vi "configure operation.vi"(7 "Shared Library Module configuration in":refnum<class "Shared Library Module configuration.lvclass">, 8 "error in":errorcluster, 10 "line item in":T1, 11 "engine configuration in":refnum<class "engine configuration.lvclass">) -> (0 "error out":errorcluster, 1 "success":bool, 2 "line item out":T1, 5 "changed":bool)   [LabVIEW 2013, in "Shared Library Module editor node.lvclass"]
doc: "Platypus Framework 1.0.1.60\nNI Systems Engineering - National Instruments"
uses:
  Shared Library Module editor node.lvclass
  permissions.ctl
  table line.ctl
  <vilib>/NI/Tag Bus Module Framework/channel/TBM channel.lvclass
  <vilib>/NI/Module Execution Interface/Engine Configuration/engine configuration.lvclass
  configuration/Shared Library Module configuration.lvclass
  <vilib>/NI/Configuration Framework/serializable configuration/NISE_CEF_serializable configuration.lvclass/NISE_CEF_serializable configuration.ctl
  <vilib>/NI/Tag Bus Module Framework/channel/TBM channel.lvclass/TBM channel.ctl
  <vilib>/NI/Tag Bus/tag/tag descriptor.lvclass/tag descriptor.ctl
  <vilib>/NI/Configuration Framework/serializable configuration/Read UID.vi
  <vilib>/NI/Tag Bus Module Framework/channel/Read channel classification.vi
  <vilib>/NI/Tag Bus/tag/read data type.vi
  <vilib>/NI/Tag Bus/tag/write tag name.vi
  <vilib>/NI/Tag Bus/tag/write data type.vi
  <vilib>/NI/Tag Bus Module Framework/channel/Write channel classification.vi
  <vilib>/Utility/LVClass/Get LV Class Name.vi
  <vilib>/NI/Configuration Framework/error generator/NISE_error generator.vi
  <vilib>/NI/Tag Bus/tag/tag descriptor.lvclass
panel:
  in  "Tag":i32(listbox)
  in  "Type":i32(listbox)
  in  "Channel Name":string
  in  "cancel":bool
  in  "ok":bool
  in  "Access Type":T2
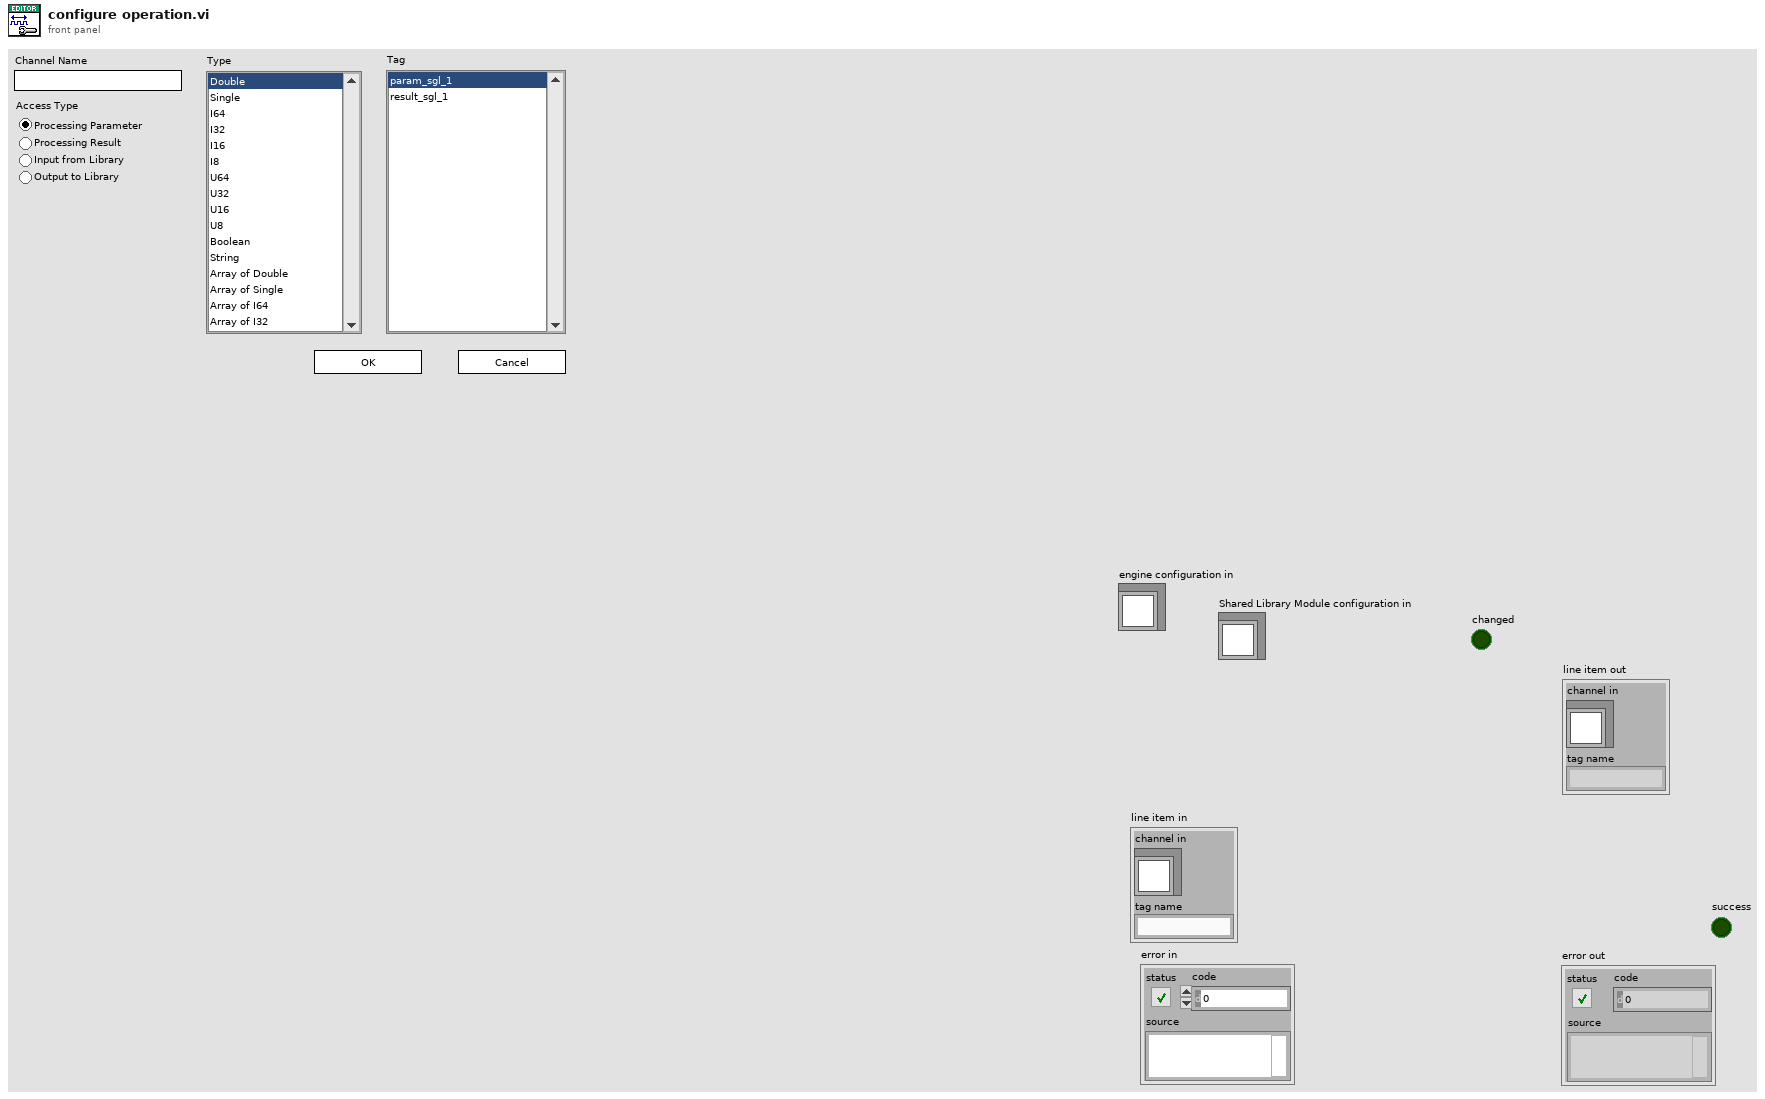
[diagram p1: front panel]
types:
  T1 = typedef "Shared Library Module editor node.lvclass/table line.ctl" = cluster{"channel in":refnum<class "TBM channel.lvclass">, "tag name":string}
  T2 = typedef "Shared Library Module editor node.lvclass/permissions.ctl" = enum32{"Processing Parameter", "Processing Result", "Input from Library", "Output to Library"}
  T3 = enum32{"Invalid", "Standard", "Closed", "Hidden", "Minimized", "Maximized"}
  T4 = enum32{"Invalid", "Default", "Floating", "Floating/Auto-Hide", "Modal"}
  T5 = enum8{"Enabled", "Disabled", "Disabled and Grayed Out"}
  T6 = typedef "tag bus.lvlib/tag descriptor.lvclass/Data Type.ctl" = enum16{"Double", "Single", "I64", "I32", "I16", "I8", "U64", "U32", "U16", "U8", "Boolean", "String", "Array of Double", "Array of Single", "Array of I64", "Array of I32", "Array of I16", "Array of I8", "Array of U64", "Array of U32", "Array of U16", "Array of U8", "Array of Boolean", "Array of String"}
  T7 = enum32{"invalid app kind", "Development System", "Run Time System", "Student Edition", "Embedded LabVIEW", "Evaluation", "Custom"}
  T8 = typedef "TBM channel.lvclass/channel classification.ctl" = enum16{"input data", "output data", "processing parameter", "processing result"}
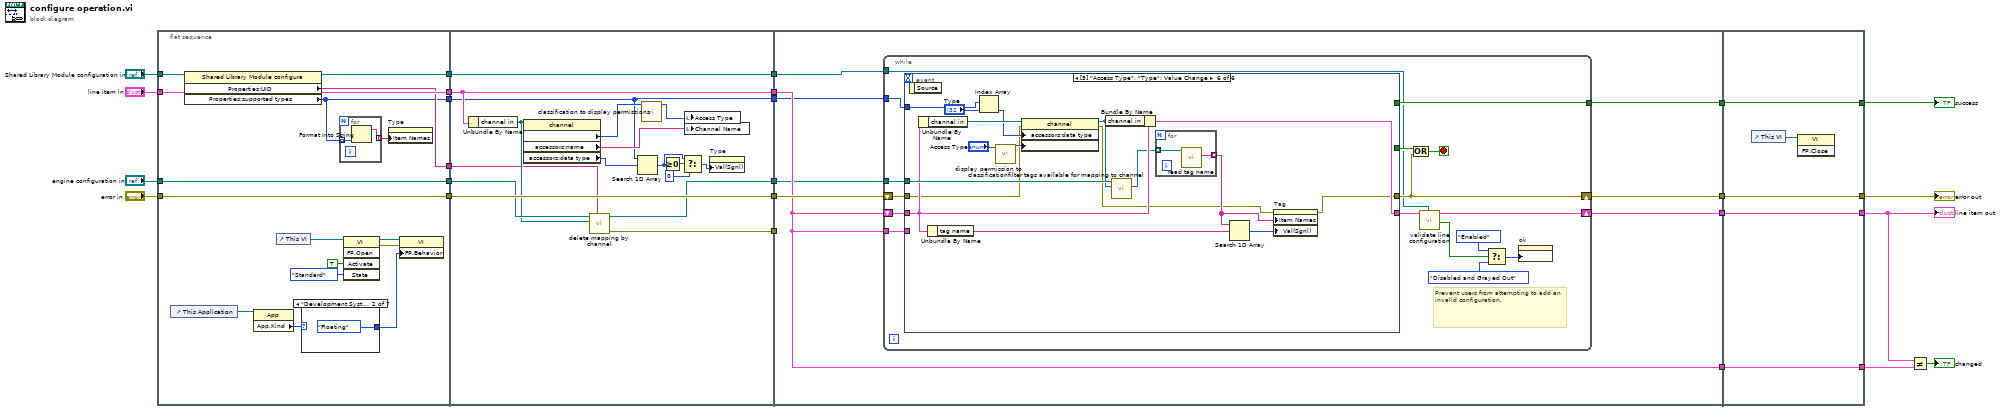
[diagram p0: block diagram]
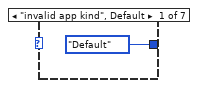
[diagram p2: hidden frame]
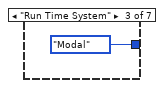
[diagram p3: hidden frame]
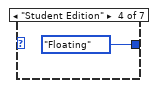
[diagram p4: hidden frame]
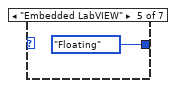
[diagram p5: hidden frame]
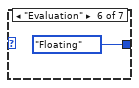
[diagram p6: hidden frame]
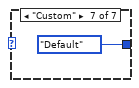
[diagram p7: hidden frame]
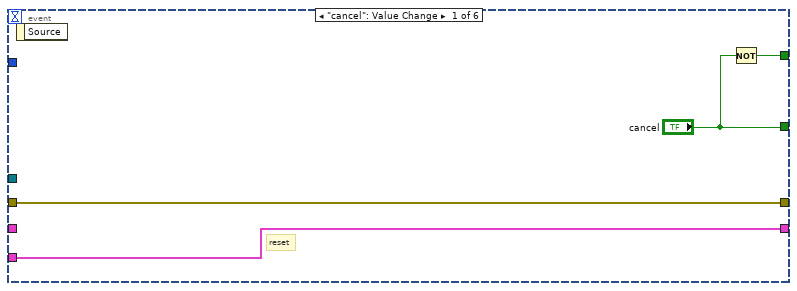
[diagram p8: hidden frame]
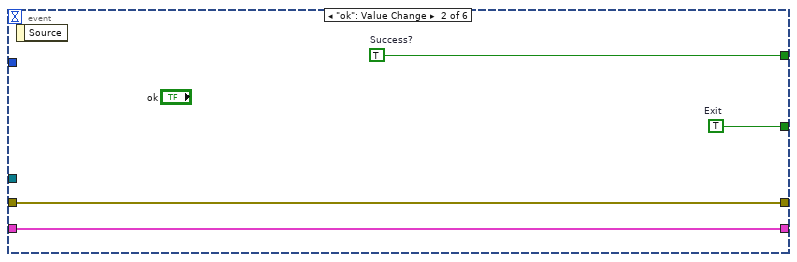
[diagram p9: hidden frame]
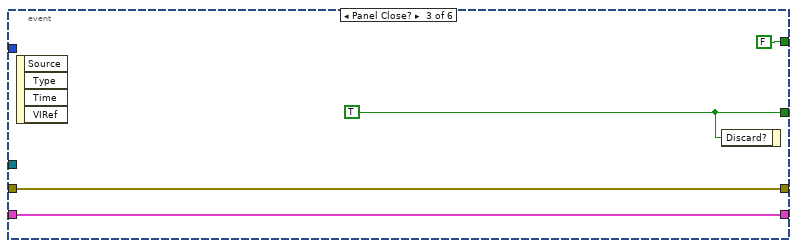
[diagram p10: hidden frame]
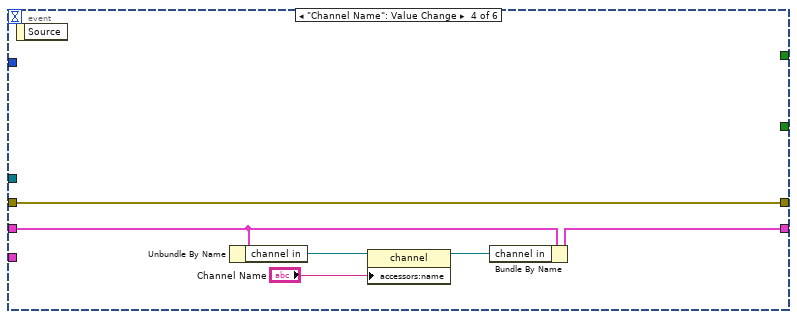
[diagram p11: hidden frame]
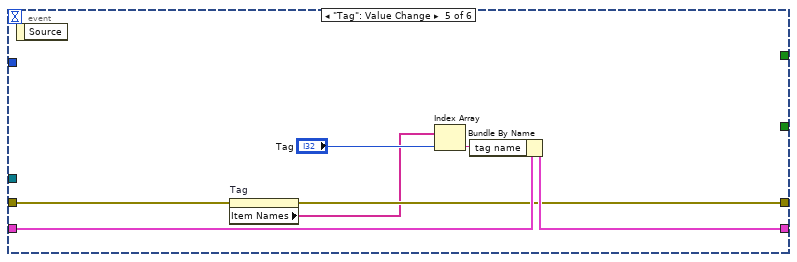
[diagram p12: hidden frame]
diagram:
  n1 = flat-sequence {
    tunnel: "line item in" -> [w40]
    tunnel: "error in" -> [w41]
    tunnel: [w41] -> w14
    tunnel: [w40] -> w12
    tunnel: [w29] -> w10
    tunnel: "Shared Library Module configuration in" -> [w31]
    tunnel: "engine configuration in" -> [w30]
    tunnel: [w30] -> w6
    tunnel: [w28] -> w4
    tunnel: [w27] -> w3
    tunnel: w14 -> [w67]
    tunnel: [w67] -> w13
    tunnel: w12 -> [w63]
    tunnel: [w63] -> w11
    tunnel: w10 -> [w62]
    tunnel: [w62] -> w8
    tunnel: w6 -> [w61]
    tunnel: [w60] -> w5
    tunnel: w4 -> [w58]
    tunnel: w3 -> [w56]
    tunnel: [w56] -> w2
    tunnel: [w51] -> w1
    tunnel: [w74] -> w18
    tunnel: [w73] -> w17
    tunnel: [w72] -> w16
    tunnel: [w71] -> w15
    tunnel: w13 -> [w75]
    tunnel: w11 -> [w71]
    tunnel: w8 -> [w70]
    tunnel: w5 -> [w69]
    tunnel: w2 -> [w68]
    tunnel: w1 -> [_]
    tunnel: [w137] -> w19
    tunnel: [w138] -> w22
    tunnel: [w139] -> w23
    tunnel: [w140] -> w24
    tunnel: w18 -> [w140]
    tunnel: w17 -> [w139]
    tunnel: w16 -> [w138]
    tunnel: w15 -> [w137]
    frame #0 {
      n2 = control-ref of="This Application"() -> (w34:refnum<vi>)
      n3 = property class="Shared Library Module configura"(reference=w31) -> (reference out=w29:refnum<class "Shared Library Module configuration.lvclass">, "Properties:UID"=w28:string, "Properties:supported types"=w27:T6[])  [unwired: 1 in, 1 out]
      n4 = property class="App"(reference=w34) -> ("App.Kind"=w33:T7)  [unwired: 1 in, 2 out]
      n5 = control-ref of="This VI"() -> (w35:refnum<vi>)
      n6 = case shown="\"Development System\"" w33 {
        tunnel: [T4."Default" ("Front Panel Window:Behavior") T4."Floating" ("Front Panel Window:Behavior") T4."Modal" ("Front Panel Window:Behavior") T4."Floating" ("Front Panel Window:Behavior") T4."Floating" ("Front Panel Window:Behavior") T4."Floating" ("Front Panel Window:Behavior") T4."Default" ("Front Panel Window:Behavior")] -> w32
        frame "invalid app kind", Default {
        }
        frame "Development System" {
        }
        frame "Run Time System" {
        }
        frame "Student Edition" {
        }
        frame "Embedded LabVIEW" {
        }
        frame "Evaluation" {
        }
        frame "Custom" {
        }
      }
      n7 = for {
        tunnel: w27 -> [w43] mode=indexing
        tunnel: [w42] -> w26 mode=indexing
        n8 = Format Into String(w43) -> (resulting string=w42:string)  [unwired: 3 in, 1 out]
      }
      n9 = invoke class="VI" method="FP.Open"(reference=w35, "Activate"=TRUE ("Activate?"), "State"=T3."Standard") -> (reference out=w38:refnum<vi>, error out=w39:errorcluster)  [unwired: 2 in, 3 out]
      n10 = property on="Type" class="LstBox (strict)"("Item Names"=w26) -> ()  [unwired: 2 in, 2 out]
      n11 = property class="VI"(reference=w38, error in=w39, "FP.Behavior"=w32) -> ()  [unwired: 2 out]
    }
    frame #1 {
      n12 = Unbundle By Name(w63) -> ("channel in"=w59:refnum<class "TBM channel.lvclass">)
      n13 = property class="channel"(reference=w59) -> ("data access:channel classification"=w66:T8, "accessors:name"=w65:string, "accessors:data type"=w57:T6)  [unwired: 1 in, 2 out]
      n14 = call <vilib>:"delete mapping by channel.vi"("owner ID"=w58, "channel"=w59, "engine configuration in"=w61) -> ("error out"=w51:errorcluster, "engine configuration out"=w60:refnum<class "engine configuration.lvclass">)  [unwired: 7 in]
      n15 = Search 1D Array(1D array=w56, element=w57) -> (index of element=w54:i32)  [unwired: 1 in]
      n16 = call "classification to display permissions.vi"("channel classification"=w66) -> ("permissions"=w64:T2)  [unwired: 10 in]
      n17 = Greater Or Equal To 0?(x=w54) -> (x >= 0?=w55:bool)
      n18 = Select(t=w54, s=w55, f=0) -> (s? t:f=w53:i32)
      n19 = local write "Access Type"(w64) -> ()
      n20 = local write "Channel Name"(w65) -> ()
      n21 = property on="Type" class="LstBox (strict)"("Val(Sgnl)"=w53) -> ()  [unwired: 2 in, 2 out]
    }
    frame #2 {
      n22 = while {
        shift-right: [w82] -> w73
        shift-left: w75 -> [w90]
        tunnel: [w89] -> w74
        shift-right: [w83] -> w72
        shift-left: w71 -> [w86]
        tunnel: w71 -> [w85]
        tunnel: w69 -> [w91]
        tunnel: w70 -> [w77]
        tunnel: w68 -> [w76]
        stop <- w87 stop-if-true
        # "Prevent users from attempting to add an invalid configuration."
        n23 = event shown="[5] \"Access Type\", \"Type\": Value Change" {
          selector: _ -> [_ _ _ _ _ _]
          dyn-events: _ -> [_ _ _ _ _ _]
          timeout: _ -> [_ _ _ _ _ _]
          tunnel: w91 -> [_ _ _ _ _ w130]
          tunnel: w90 -> [w95 w99 w103 w109 w112 w119]
          tunnel: [w95 w99 w103 w109 w111 w117] -> w82
          tunnel: [w94 w96 FALSE _ _ _] -> w89
          tunnel: ["cancel" w97 w101 _ _ _] -> w88
          tunnel: w86 -> [_ w98 w100 w107 w116 w128]
          tunnel: [w92 w98 w100 w108 w115 w127] -> w84
          tunnel: w85 -> [w92 _ _ _ _ _]
          tunnel: w76 -> [_ _ _ _ _ w125]
          event "cancel": Value Change {
            # "reset"
            n24 = event-data() -> ()  [unwired: 1 in, 1 out]
            n25 = Not(x="cancel") -> (.not. x?=w94:bool)
          }
          event "ok": Value Change {
            w96 = TRUE  # Success?
            w97 = TRUE  # Exit
            n26 = event-data() -> ()  [unwired: 1 in, 1 out]
          }
          event Panel Close? {
            w101 = TRUE ("cancel")
            n27 = event-data() -> ()  [unwired: 1 in, 4 out]
            n28 = event-data("Discard?"=w101) -> ()  [unwired: 1 in, 1 out]
          }
          event "Channel Name": Value Change {
            n29 = event-data() -> ()  [unwired: 1 in, 1 out]
            n30 = Unbundle By Name(w107) -> ("channel in"=w106:refnum<class "TBM channel.lvclass">)
            n31 = property class="channel"(reference=w106, "accessors:name"="Channel Name") -> (reference out=w105:refnum<class "TBM channel.lvclass">)  [unwired: 1 in, 1 out]
            n32 = Bundle By Name(cluster=w107, "channel in"=w105) -> (w108:T1)
          }
          event "Tag": Value Change {
            n33 = event-data() -> ()  [unwired: 1 in, 1 out]
            n34 = property on="Tag" class="LstBox (strict)"(error in=w112) -> (error out=w111:errorcluster, "Item Names"=w110:string[])  [unwired: 1 in, 1 out]
            n35 = Index Array(array=w110, index="Tag") -> (element=w114:string)
            n36 = Bundle By Name(cluster=w116, "tag name"=w114) -> (w115:T1)
          }
          event "Type": Value Change {
            n37 = event-data() -> ()  [unwired: 1 in, 1 out]
            n38 = Unbundle By Name(w128) -> ("channel in"=w132:refnum<class "TBM channel.lvclass">)
            n39 = Unbundle By Name(w128) -> ("tag name"=w122:string)
            n40 = Index Array(array=w125, index="Type") -> (element=w123:T6)
            n41 = call "display permission to classification.vi"("display permissions"="Access Type") -> ("channel classification"=w131:T8)  [unwired: 10 in]
            n42 = property class="channel"(reference=w132, error in=w119, "accessors:data type"=w123, "data access:channel classification"=w131) -> (reference out=w129:refnum<class "TBM channel.lvclass">, error out=w118:errorcluster)
            n43 = Bundle By Name(cluster=w128, "channel in"=w129) -> (w127:T1)
            n44 = call <vilib>:"filter tags available for mapping to channel.vi"("channel to map to"=w129, "engine configuration in"=w130) -> ("filtered tags"=w126:refnum<class "tag descriptor.lvclass">[])  [unwired: 8 in, 1 out]
            n45 = for {
              tunnel: w126 -> [w135] mode=indexing
              tunnel: [w134] -> w120 mode=indexing
              n46 = call <vilib>:"read tag name.vi"("system tag in"=w135) -> ("name"=w134:string)  [unwired: 8 in, 2 out]
            }
            n47 = Search 1D Array(1D array=w120, element=w122) -> (index of element=w121:i32)  [unwired: 1 in]
            n48 = property on="Tag" class="LstBox (strict)"(error in=w118, "Item Names"=w120, "Val(Sgnl)"=w121) -> (error out=w117:errorcluster)  [unwired: 1 in, 1 out]
          }
        }
        n49 = Compound Arithmetic op=OR(w88, w82) -> (w87:bool)
        n50 = call "validate line configuration.vi"("module configuration"=w77, "line in"=w84) -> ("valid?"=w81:bool, "line out"=w83:T1)  [unwired: 8 in]
        n51 = Select(t=T5."Enabled" ("Disabled"), s=w81, f=T5."Disabled and Grayed Out") -> (s? t:f=w78:T5)
        n52 = property on="ok" class="Bool"("DisabledEnum"=w78) -> ()  [unwired: 2 in, 2 out]
      }
    }
    frame #3 {
      n53 = control-ref of="This VI"() -> (w136:refnum<vi>)
      n54 = invoke class="VI" method="FP.Close"(reference=w136) -> ()  [unwired: 2 in, 3 out]
    }
  }
  n55 = Not Equal?(x=w22, y=w19) -> (x != y?=→"changed":bool)
  "error out" <- w23
  "success" <- w24
  "line item out" <- w22
